vi "LoadParser.vi"(4 "PythonPath":path, 5 "SessionName":string, 6 "PythonVersion":string, 7 "ModulePath":path, 8 "error in (no error)":errorcluster, 9 "ParserName":string, 10 "ParserPath":path, 11 "ArgumentParser in":refnum<class "ArgumentParser.lvclass">) -> (0 "error out":errorcluster, 3 "ArgumentParser out":refnum<class "ArgumentParser.lvclass">)   [LabVIEW 2022 SP3, in "ArgumentParser.lvlib" / "ArgumentParser.lvclass"]
uses:
  ArgumentParser.lvclass
  C:/Users/jakub/repos/gh/sw4sys/lv-argument-parser/PythonWrapper/Source/PythonSession/PythonSession.lvclass
  C:/Users/jakub/repos/gh/sw4sys/lv-argument-parser/PythonWrapper/Source/PythonWrapper/PythonWrapper.lvclass
  C:/Users/jakub/repos/gh/sw4sys/lv-argument-parser/ArgumentParser/Source/ArgparseWrapper/ArgparseWrapper.lvclass
  PythonWrapper/Source/PythonSession/PythonSession.lvclass/PythonSession.ctl
  PythonWrapper/Source/PythonWrapper/PythonWrapper.lvclass/PythonWrapper.ctl
  ArgumentParser.lvclass/ArgumentParser.ctl
  ArgparseWrapper/ArgparseWrapper.lvclass/ArgparseWrapper.ctl
  PythonWrapper/Source/PythonSession/Write SessionName.vi
  PythonWrapper/Source/PythonSession/Write PythonVersion.vi
  PythonWrapper/Source/PythonSession/Write PythonPath.vi
  PythonWrapper/Source/PythonWrapper/Write ModulePath.vi
  Write ParserPath.vi
  PythonWrapper/Source/PythonSession/Read PythonSession.vi
  PythonWrapper/Source/PythonWrapper/Read ModulePath.vi
  Read ParserPath.vi
  Write ParserName.vi
  PythonWrapper/Source/PythonSession/SessionBank.vi
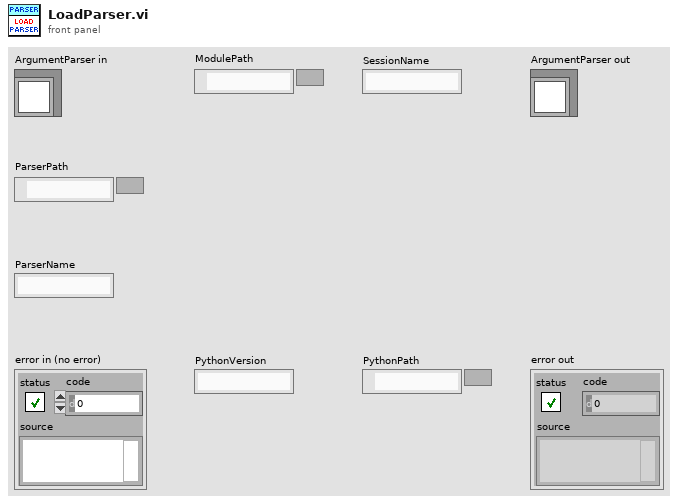
[diagram p1: front panel]
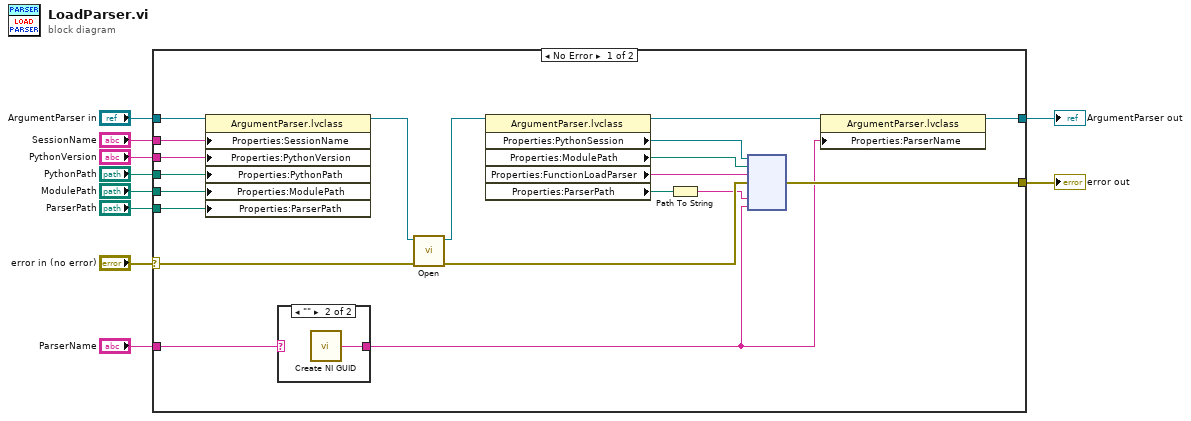
[diagram p0: block diagram]
diagram:
  n1 = case shown="No Error" "error in (no error)" {
    selector: "error in (no error)" -> [w29 w34]
    tunnel: [w30 w34] -> w9
    tunnel: [w28 w33] -> w8
    tunnel: "ModulePath" -> [w18 _]
    tunnel: "ParserPath" -> [w22 _]
    tunnel: "PythonVersion" -> [w20 _]
    tunnel: "PythonPath" -> [w19 _]
    tunnel: "SessionName" -> [w17 _]
    tunnel: "ParserName" -> [w14 _]
    tunnel: "ArgumentParser in" -> [w11 w33]
    frame No Error {
      n2 = property class="ArgumentParser.lvclass"(reference=w11, "Properties:SessionName"=w17, "Properties:PythonVersion"=w20, "Properties:PythonPath"=w19, "Properties:ModulePath"=w18, "Properties:ParserPath"=w22) -> (reference out=w16:refnum<class "ArgumentParser.lvclass">)  [unwired: 1 in, 1 out]
      n3 = case shown="\"\"" w14 {
        selector: w14 -> [w31 _]
        tunnel: [w31 w32] -> w13
        frame Default {
        }
        frame "" {
          n4 = call <vilib>:"Create NI GUID.vi"() -> ("NI GUID"=w32:string)
        }
      }
      n5 = call-dynamic "Open.vi"("error in (no error)"=w29, "ArgumentParser in"=w16) -> ("error out"=w23:errorcluster, "ArgumentParser out"=w15:refnum<class "ArgumentParser.lvclass">)  [unwired: 8 in]
      n6 = property class="ArgumentParser.lvclass"(reference=w15) -> (reference out=w27:refnum<class "ArgumentParser.lvclass">, "Properties:PythonSession"=w25:refnum<k35>, "Properties:ModulePath"=w24:path, "Properties:FunctionLoadParser"=w26:string, "Properties:ParserPath"=w12:path)  [unwired: 1 in, 1 out]
      n7 = Path To String(path=w12) -> (string=w21:string)
      n8 = node(w25, w24, w26, w23, w21, w13) -> (w30:errorcluster)  [unwired: 4 in, 3 out]
      n9 = property class="ArgumentParser.lvclass"(reference=w27, "Properties:ParserName"=w13) -> (reference out=w28:refnum<class "ArgumentParser.lvclass">)  [unwired: 1 in, 1 out]
    }
    frame Error {
    }
  }
  "error out" <- w9
  "ArgumentParser out" <- w8
